vi "Global_count_var.vi"() -> ()   [LabVIEW 2019]
panel:
  in  "Global count":dbl
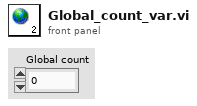
[diagram p1: front panel]
diagram:
